vi "Setup UI.vi"(8 "error in (no error)":errorcluster, 10 "Set UI to input? (F)":bool, 11 "Magnetic Field Lakeshore Scan in":refnum<class "Magnetic Field Lakeshore Scan.lvclass">) -> (0 "error out":errorcluster, 3 "Magnetic Field Lakeshore Scan out":refnum<class "Magnetic Field Lakeshore Scan.lvclass">)   [LabVIEW 2023, in "Magnetic Field Lakeshore Scan.lvclass"]
doc: "Scanner::Setup is a constructor that has no parameters and faces the user. The Factory calls this VI to let the user configure this Scanner. It is dynamically dispatched in order to let the user choose the type as well as the options of the scanner."
uses:
  Magnetic Field Lakeshore Scan.lvclass
  Magnetic Field Lakeshore Scan.lvclass/Magnetic Field Lakeshore Scan.ctl
  Instruments/Utility Classes/Scannable/Scannable.lvclass
panel:
  in  "Go to setpoint set":bool
  in  "Setpoint Set":dbl[unit]
  out "Current Setpoint":dbl[unit]
  in  "Field control on/off toggle":bool
  in  "Control slope limit":dbl[unit]=0.16666666666666666
  in  "Ramp rate":dbl[unit]=0.005833333333333334
  in  "Integral":dbl[unit]=1.0
  in  "Proportional":dbl=10.0
  in  "Field reading":dbl[unit]
  in  "Go to first point (can't see it change!)":bool
  # "Magnetic Field Lakeshore Scan Setup"
  # "Note: Independent Variable above must be given in gauss."
  # "This needs to be on before you do the \nscan or select \"Go to first point\"!"
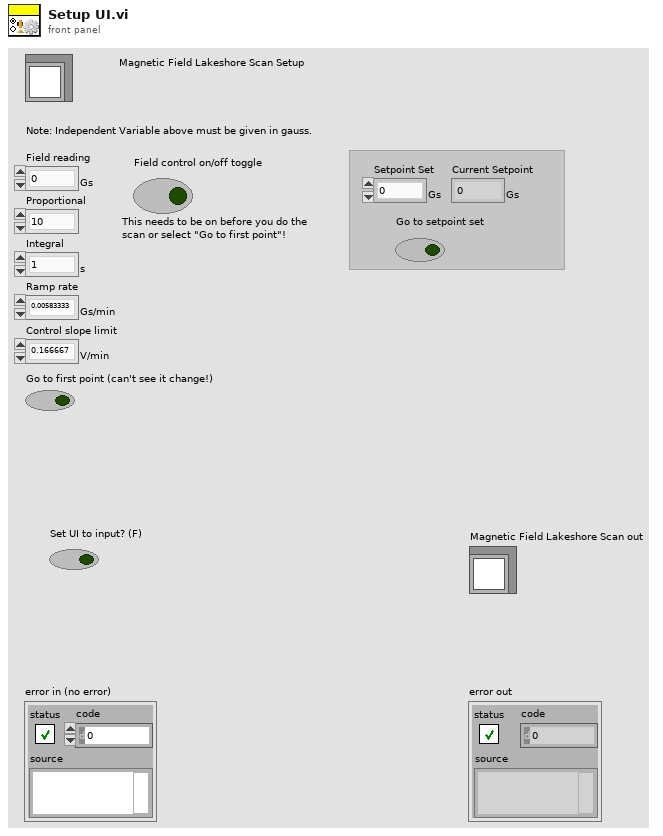
[diagram p1: front panel]
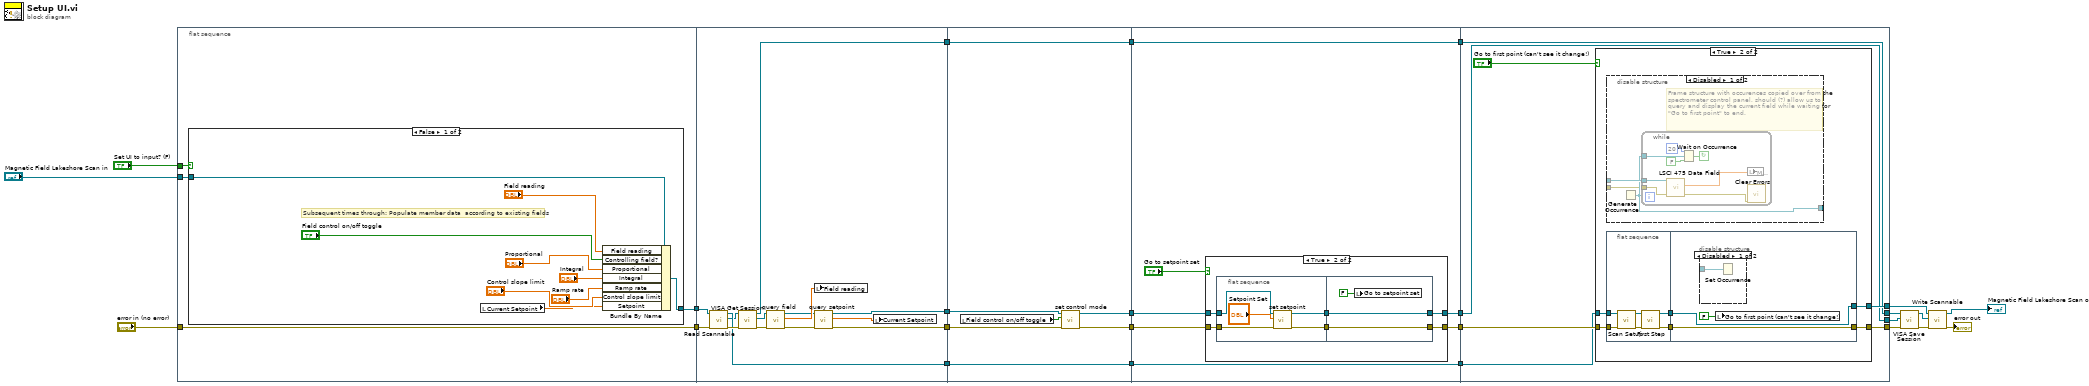
[diagram p0: block diagram]
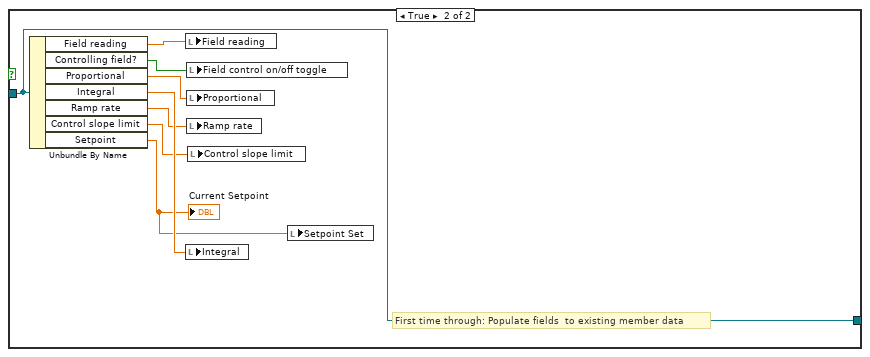
[diagram p2: hidden frame]
diagram:
  n1 = flat-sequence {
    tunnel: "Magnetic Field Lakeshore Scan in" -> [w28]
    tunnel: [w29] -> w22
    tunnel: "error in (no error)" -> [w29]
    tunnel: [w26] -> w21
    tunnel: "Set UI to input? (F)" -> [w27]
    tunnel: w22 -> [w57]
    tunnel: [w48] -> w12
    tunnel: w21 -> [w59]
    tunnel: [w58] -> w11
    tunnel: [w50] -> w10
    tunnel: [w55] -> w9
    tunnel: w12 -> [w64]
    tunnel: [w61] -> w8
    tunnel: w11 -> [w67]
    tunnel: [w67] -> w6
    tunnel: w10 -> [w63]
    tunnel: [w62] -> w4
    tunnel: w9 -> [w66]
    tunnel: [w66] -> w2
    tunnel: w8 -> [w69]
    tunnel: [w68] -> w7
    tunnel: w6 -> [w74]
    tunnel: [w74] -> w5
    tunnel: w4 -> [w71]
    tunnel: [w70] -> w3
    tunnel: w2 -> [w73]
    tunnel: [w73] -> w1
    tunnel: [w94] -> w18
    tunnel: w7 -> [w95]
    tunnel: [w96] -> w13
    tunnel: w5 -> [w92]
    tunnel: [w91] -> w20
    tunnel: w3 -> [w91]
    tunnel: [w93] -> w19
    tunnel: w1 -> [w93]
    frame #0 {
      n2 = case shown="False" w27 {
        tunnel: w28 -> [w38 w46]
        tunnel: [w37 w46] -> w26
        frame False {
          # "Subsequent times through: Populate member data  according to existing fields"
          n3 = local read "Current Setpoint"() -> (w30:dbl[unit])
          n4 = Bundle By Name(cluster=w38, "Field reading"="Field reading", "Controlling field?"="Field control on/off toggle", "Proportional"="Proportional", "Integral"="Integral", "Ramp rate"="Ramp rate", "Control slope limit"="Control slope limit", "Setpoint"=w30) -> (w37:refnum<class "Magnetic Field Lakeshore Scan.lvclass">)
        }
        frame True {
          # "First time through: Populate fields  to existing member data"
          n5 = Unbundle By Name(w46) -> ("Field reading"=w45:dbl[unit], "Controlling field?"=w40:bool, "Proportional"=w44:dbl, "Integral"=w43:dbl[unit], "Ramp rate"=w42:dbl[unit], "Control slope limit"=w41:dbl[unit], "Setpoint"=w39:dbl[unit])
          "Current Setpoint" <- w39
          n6 = local write "Field reading"(w45) -> ()
          n7 = local write "Integral"(w43) -> ()
          n8 = local write "Field control on/off toggle"(w40) -> ()
          n9 = local write "Proportional"(w44) -> ()
          n10 = local write "Ramp rate"(w42) -> ()
          n11 = local write "Control slope limit"(w41) -> ()
          n12 = local write "Setpoint Set"(w39) -> ()
        }
      }
    }
    frame #1 {
      n13 = call-dynamic "Read Scannable.vi"("error in (no error)"=w57, "Scanner.lvclass in"=w59) -> ("error out"=w60:errorcluster, "Scannable.lvclass"=w56:refnum<class "Scannable.lvclass">, "Scanner.lvclass out"=w58:refnum<class "Magnetic Field Lakeshore Scan.lvclass">)  [unwired: 7 out]
      n14 = call-dynamic "VISA Get Session.vi"("error in (no error)"=w60, "Instrument.lvclass in"=w56) -> ("error out"=w53:errorcluster, "VISA Resource Name"=w54:refnum<visa-resource-name>, "Instrument.lvclass out"=w55:refnum<class "Scannable.lvclass">)  [unwired: 7 out]
      n15 = call "query field.vi"("error in (no error)"=w53, "VISA session"=w54) -> ("error out"=w49:errorcluster, "Field reading"=w52:dbl[unit], "dup VISA session"=w51:refnum<visa-resource-name>)  [unwired: 7 in]
      n16 = local write "Field reading"(w52) -> ()
      n17 = call "query setpoint.vi"("error in (no error)"=w49, "VISA session"=w51) -> ("error out"=w48:errorcluster, "Setpoint"=w47:dbl[unit], "dup VISA session"=w50:refnum<visa-resource-name>)  [unwired: 7 in]
      n18 = local write "Current Setpoint"(w47) -> ()
    }
    frame #2 {
      n19 = local read "Field control on/off toggle"() -> (w65:bool)
      n20 = call "set control mode.vi"("error in (no error)"=w64, "Start/stop controlling field"=w65, "VISA session"=w63) -> ("error out"=w61:errorcluster, "dup VISA session"=w62:refnum<visa-resource-name>)  [unwired: 7 in]
    }
    frame #3 {
      n21 = case shown="True" "Go to setpoint set" {
        tunnel: w71 -> [w75 w82]
        tunnel: [w75 w80] -> w70
        tunnel: w69 -> [w76 w81]
        tunnel: [w76 w78] -> w68
        frame False {
        }
        frame True {
          n22 = flat-sequence {
            tunnel: w82 -> [w86]
            tunnel: w81 -> [w85]
            tunnel: [w84] -> w79
            tunnel: [w83] -> w77
            tunnel: [w89] -> w80
            tunnel: w79 -> [w89]
            tunnel: [w88] -> w78
            tunnel: w77 -> [w88]
            frame #0 {
              n23 = call "set setpoint.vi"("error in (no error)"=w85, "Setpoint"="Setpoint Set", "VISA session"=w86) -> ("error out"=w83:errorcluster, "dup VISA session"=w84:refnum<visa-resource-name>)  [unwired: 7 in]
            }
            frame #1 {
              n24 = local write "Go to setpoint set"(FALSE ("Go to setpoint set")) -> ()
            }
          }
        }
      }
    }
    frame #4 {
      n25 = case shown="True" "Go to first point (can't see it change!)" {
        tunnel: w92 -> [w99 w105]
        tunnel: [w99 w104] -> w96
        tunnel: w95 -> [w98 w100]
        tunnel: [w98 w103] -> w94
        frame False {
        }
        frame True {
          n26 = disable-structure shown="Disabled" {
            disable-tunnel: _ -> [w108 _]
            disable-tunnel: [w107 _] -> _
            disable-tunnel: _ -> [w106 _]
            frame Disabled {
              # "Frame structure with occurences copied over from the spectrometer control panel, should (?) allow us to query and display the current field while waiting for \"Go to first point\" to end."
              n27 = Generate Occurrence() -> (w107:refnum<k4>)
              n28 = while {
                tunnel: w107 -> [w113]
                tunnel: w108 -> [w111]
                tunnel: w106 -> [w110]
                stop <- w112 continue-if-true
                n29 = call "LSCI 475 Data Field.vi"("error in (no error)"=w110, "VISA session"=w111) -> ("error out"=w109:errorcluster, "Field Reading"=w116:dbl)  [unwired: 7 in, 1 out]
                n30 = Wait on Occurrence(1:FALSE ("ignore previous (T)"), 2:w113, 3:20 ("ms timeout (-1)")) -> (0:w112:bool)
                n31 = local write item#-1(w116) -> ()
                n32 = call <vilib>:"Clear Errors.vi"("error in (no error)"=w109) -> ()  [unwired: 1 in, 6 out]
              }
            }
            frame Enabled {
            }
          }
          n33 = flat-sequence {
            tunnel: w105 -> [w122]
            tunnel: w100 -> [w119]
            tunnel: [w120] -> w102
            tunnel: [w117] -> w101
            tunnel: [w124] -> w103
            tunnel: [w125] -> w104
            tunnel: w102 -> [w125]
            tunnel: w101 -> [w124]
            frame #0 {
              n34 = call-dynamic "Scan Setup.vi"("error in (no error)"=w119, "Magnetic Field Lakeshore Scan in"=w122) -> ("error out"=w118:errorcluster, "Magnetic Field Lakeshore Scan out"=w121:refnum<class "Magnetic Field Lakeshore Scan.lvclass">)  [unwired: 8 in]
              n35 = call-dynamic "First Step.vi"("error in (no error)"=w118, "Magnetic Field Lakeshore Scan.lvclass in"=w121) -> ("error out"=w117:errorcluster, "Magnetic Field Lakeshore Scan.lvclass out"=w120:refnum<class "Magnetic Field Lakeshore Scan.lvclass">)  [unwired: 7 in, 1 out]
            }
            frame #1 {
              n36 = disable-structure shown="Disabled" {
                disable-tunnel: _ -> [w126 _]
                frame Disabled {
                  n37 = Set Occurrence(w126) -> ()
                }
                frame Enabled {
                }
              }
              n38 = local write "Go to first point (can't see it change!)"(FALSE ("Go to first point")) -> ()
            }
          }
        }
      }
    }
  }
  n39 = call-dynamic "VISA Save Session.vi"("error in (no error)"=w18, "VISA Resource Name"=w20, "Instrument.lvclass in"=w19) -> ("error out"=w17:errorcluster, "Instrument.lvclass out"=w15:refnum<class "Scannable.lvclass">)  [unwired: 7 out]
  n40 = call-dynamic "Write Scannable.vi"("error in (no error)"=w17, "Scannable.lvclass"=w15, "Scanner.lvclass in"=w13) -> ("error out"=→"error out":errorcluster, "Scanner.lvclass out"=→"Magnetic Field Lakeshore Scan out":refnum<class "Magnetic Field Lakeshore Scan.lvclass">)  [unwired: 7 out]
